vi "picross-complete.vi"() -> ()   [LabVIEW 2020]
panel:
  out "Top":string[](array[string])
  out "Left":string[](array[string])
  out "2D Picture 100":picture
  out "2D Picture 99":picture
  out "2D Picture 98":picture
  out "2D Picture 97":picture
  out "2D Picture 96":picture
  out "2D Picture 95":picture
  out "2D Picture 94":picture
  out "2D Picture 93":picture
  out "2D Picture 92":picture
  out "2D Picture 91":picture
  out "2D Picture 90":picture
  out "2D Picture 89":picture
  out "2D Picture 88":picture
  out "2D Picture 87":picture
  out "2D Picture 86":picture
  out "2D Picture 85":picture
  out "2D Picture 84":picture
  out "2D Picture 83":picture
  out "2D Picture 82":picture
  out "2D Picture 81":picture
  out "2D Picture 80":picture
  out "2D Picture 79":picture
  out "2D Picture 78":picture
  out "2D Picture 77":picture
  out "2D Picture 76":picture
  out "2D Picture 75":picture
  out "2D Picture 74":picture
  out "2D Picture 73":picture
  out "2D Picture 72":picture
  out "2D Picture 71":picture
  out "2D Picture 70":picture
  out "2D Picture 69":picture
  out "2D Picture 68":picture
  out "2D Picture 67":picture
  out "2D Picture 66":picture
  out "2D Picture 65":picture
  out "2D Picture 64":picture
  out "2D Picture 63":picture
  out "2D Picture 62":picture
  out "2D Picture 61":picture
  out "2D Picture 60":picture
  out "2D Picture 59":picture
  out "2D Picture 58":picture
  out "2D Picture 57":picture
  out "2D Picture 56":picture
  out "2D Picture 55":picture
  out "2D Picture 54":picture
  out "2D Picture 53":picture
  out "2D Picture 52":picture
  out "2D Picture 51":picture
  out "2D Picture 50":picture
  out "2D Picture 49":picture
  out "2D Picture 48":picture
  out "2D Picture 47":picture
  out "2D Picture 46":picture
  out "2D Picture 45":picture
  out "2D Picture 44":picture
  out "2D Picture 43":picture
  out "2D Picture 42":picture
  out "2D Picture 41":picture
  out "2D Picture 40":picture
  out "2D Picture 39":picture
  out "2D Picture 38":picture
  out "2D Picture 37":picture
  out "2D Picture 36":picture
  out "2D Picture 35":picture
  out "2D Picture 34":picture
  out "2D Picture 33":picture
  out "2D Picture 32":picture
  out "2D Picture 31":picture
  out "2D Picture 30":picture
  out "2D Picture 29":picture
  out "2D Picture 28":picture
  out "2D Picture 27":picture
  out "2D Picture 26":picture
  out "2D Picture 25":picture
  out "2D Picture 24":picture
  out "2D Picture 23":picture
  out "2D Picture 22":picture
  out "2D Picture 21":picture
  out "2D Picture 20":picture
  out "2D Picture 19":picture
  out "2D Picture 18":picture
  out "2D Picture 17":picture
  out "2D Picture 16":picture
  out "2D Picture 15":picture
  out "2D Picture 14":picture
  out "2D Picture 13":picture
  out "2D Picture 12":picture
  out "2D Picture 11":picture
  out "2D Picture 10":picture
  out "2D Picture 9":picture
  out "2D Picture 8":picture
  out "2D Picture 7":picture
  out "2D Picture 6":picture
  out "2D Picture 5":picture
  out "2D Picture 4":picture
  out "2D Picture 3":picture
  out "2D Picture 2":picture
  out "2D Picture":picture
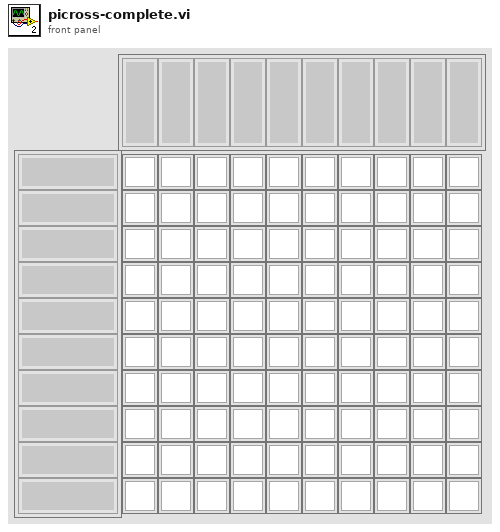
[diagram p1: front panel]
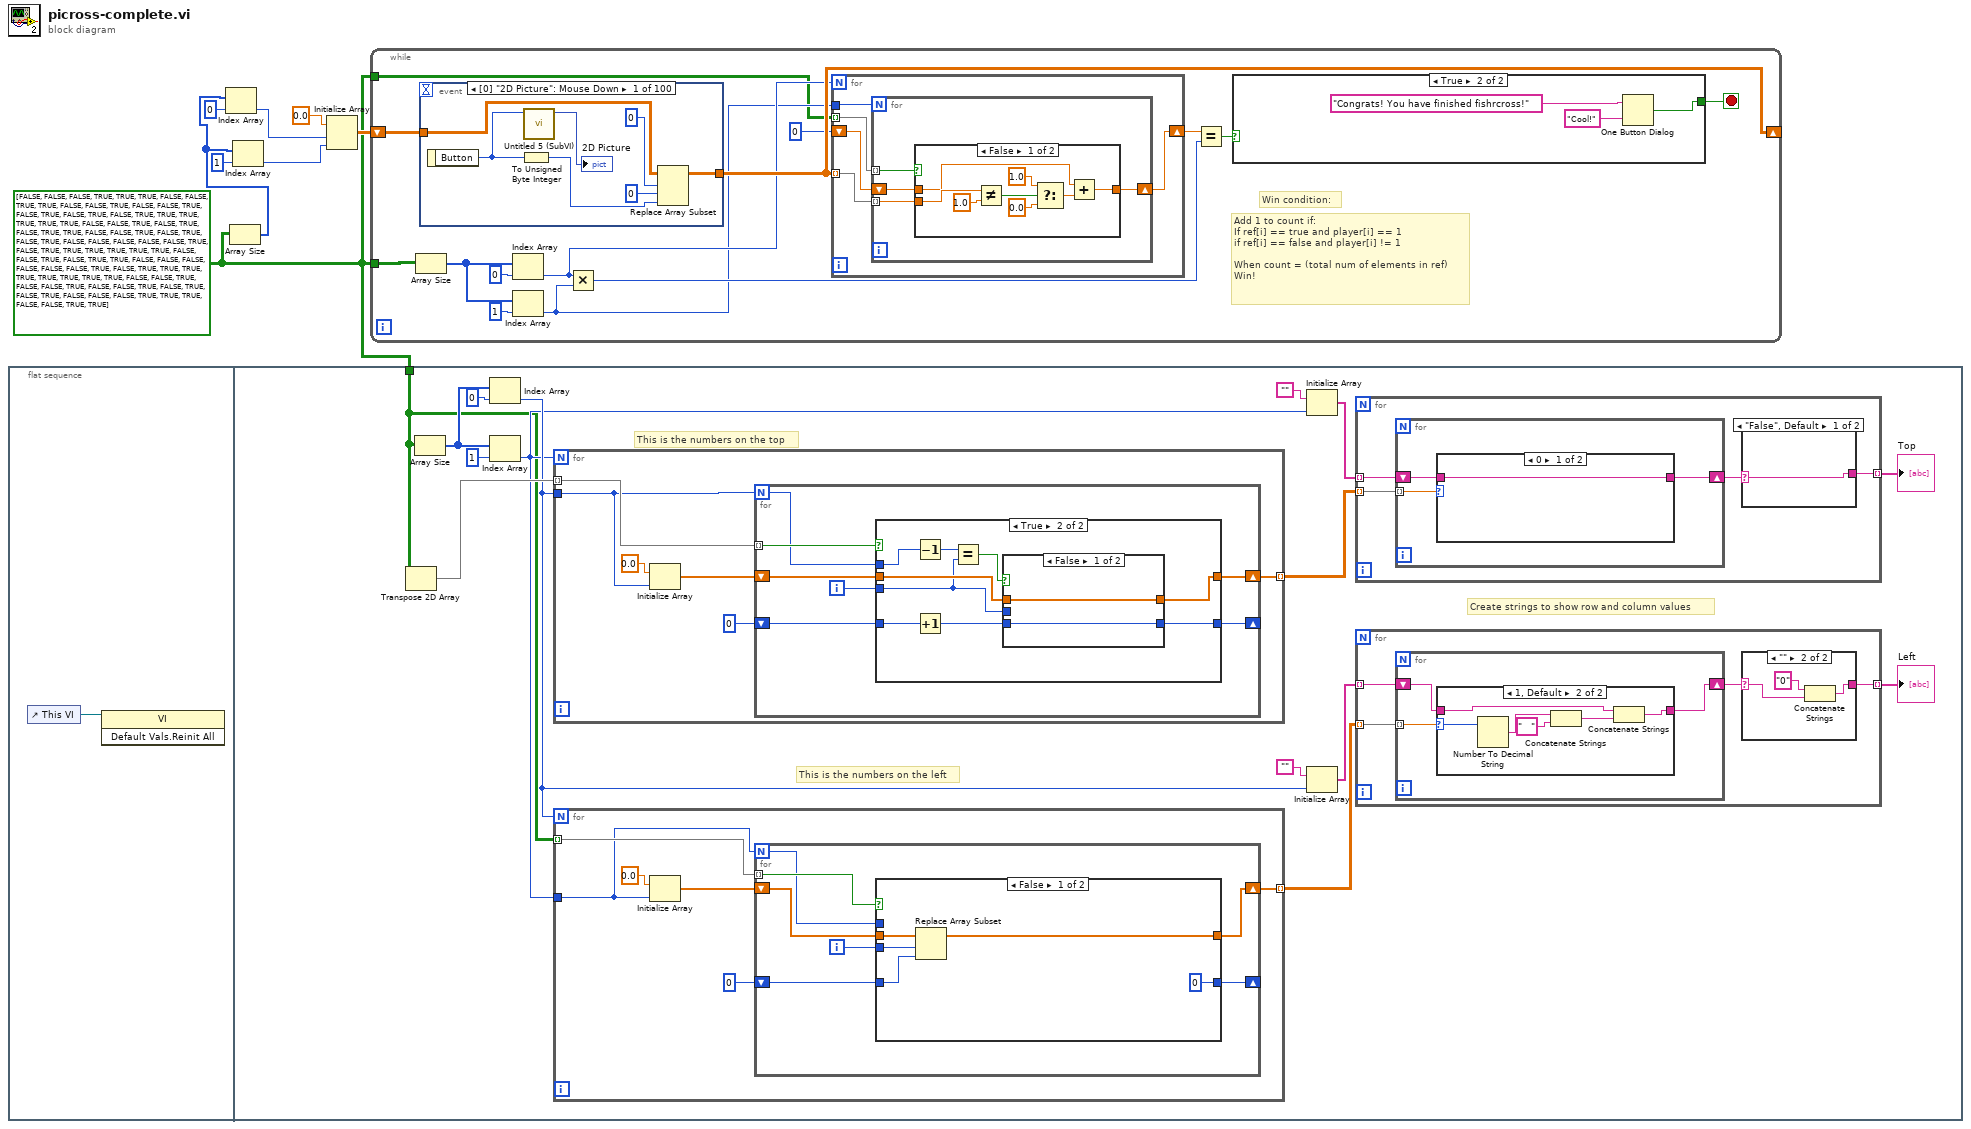
[diagram p0: block diagram]
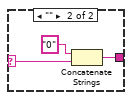
[diagram p2: hidden frame]
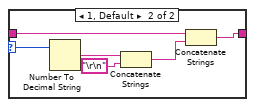
[diagram p3: hidden frame]
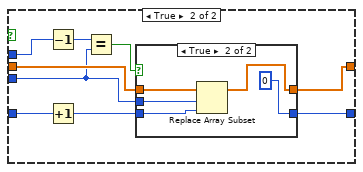
[diagram p6: hidden frame]
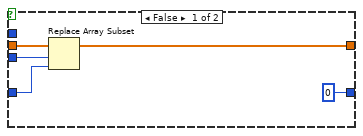
[diagram p8: hidden frame]
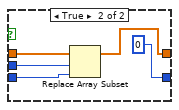
[diagram p9: hidden frame]
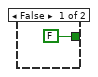
[diagram p10: hidden frame]
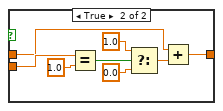
[diagram p11: hidden frame]
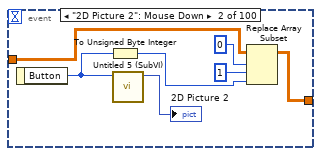
[diagram p12: hidden frame]
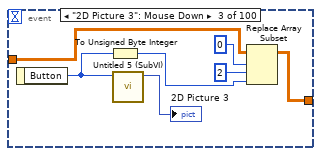
[diagram p13: hidden frame]
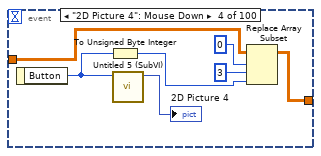
[diagram p14: hidden frame]
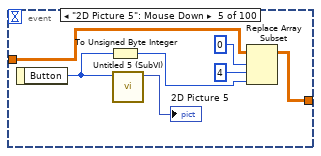
[diagram p15: hidden frame]
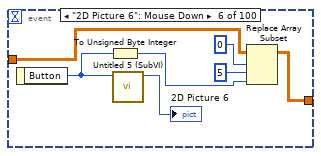
[diagram p16: hidden frame]
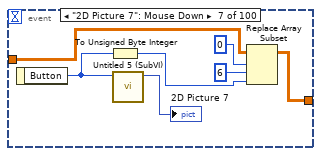
[diagram p17: hidden frame]
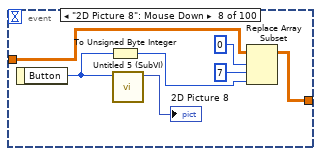
[diagram p18: hidden frame]
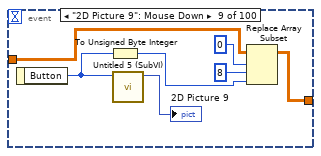
[diagram p19: hidden frame]
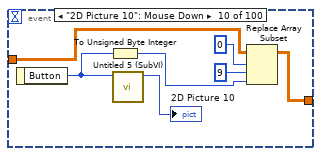
[diagram p20: hidden frame]
diagram:
  w3 = bool[][] [[FALSE, FALSE, FALSE, TRUE, TRUE, TRUE, FALSE, FALSE, TRUE, TRUE], [FALSE, FALSE, TRUE, FALSE, FALSE, TRUE, FALSE, TRUE, FALSE, TRUE], [FALSE, TRUE, TRUE, TRUE, TRUE, TRUE, TRUE, FALSE, FALSE, TRUE], [FALSE, TRUE, FALSE, TRUE, TRUE, FALSE, FALSE, TRUE, FALSE, TRUE], [FALSE, TRUE, FALSE, FALSE, FALSE, FALSE, FALSE, TRUE, FALSE, TRUE], [TRUE, TRUE, TRUE, TRUE, TRUE, FALSE, FALSE, TRUE, FALSE, TRUE], [TRUE, FALSE, FALSE, FALSE, FALSE, FALSE, FALSE, TRUE, FALSE, TRUE], [TRUE, TRUE, TRUE, TRUE, TRUE, TRUE, TRUE, FALSE, FALSE, TRUE], [FALSE, FALSE, TRUE, FALSE, FALSE, TRUE, FALSE, TRUE, FALSE, TRUE], [FALSE, FALSE, FALSE, TRUE, TRUE, TRUE, FALSE, FALSE, TRUE, TRUE]]
  n1 = flat-sequence {
    tunnel: w3 -> [w10]
    frame #0 {
      n2 = control-ref of="This VI"() -> (w9:refnum<vi>)
      n3 = invoke class="VI" method="Default Vals.Reinit All"(reference=w9) -> ()  [unwired: 2 in, 3 out]
    }
    frame #1 {
      # "Create strings to show row and column values"
      # "This is the numbers on the top"
      # "This is the numbers on the left"
      n4 = Transpose 2D Array(2D array=w10) -> (transposed array=w24:bool[][])
      n5 = Array Size(array=w10) -> (size(s)=w23:i32[])
      n6 = Index Array(array=w23, index=0) -> (element=w19:i32)
      n7 = Index Array(array=w23, index=1) -> (element=w14:i32)
      n8 = for {
        N: w14 -> [_]
        tunnel: w19 -> [w95]
        tunnel: w24 -> [w100] mode=indexing
        tunnel: [w96] -> w12 mode=indexing
        n9 = Initialize Array(0.0 ("element"), w95) -> (w97:dbl[])
        n10 = for {
          N: w95 -> [w101]
          tunnel: w100 -> [w107] mode=indexing
          shift-right: [w103] -> w96
          shift-left: w97 -> [w106]
          shift-right: [w104] -> _
          shift-left: 0 -> [w105]
          i -> [w102]
          n11 = case shown="True" w107 {
            tunnel: w106 -> [w111 w114]
            tunnel: w105 -> [w112 w121]
            tunnel: [0 w116] -> w104
            tunnel: [w110 w115] -> w103
            tunnel: w102 -> [w108 w113]
            tunnel: w101 -> [_ w120]
            frame False {
              n12 = Replace Array Subset(array=w111, new element=w112, index=w108) -> (w110:dbl[])
            }
            frame True {
              n13 = Decrement(x=w120) -> (x-1=w119:i32)
              n14 = Increment(x=w121) -> (x+1=w117:i32)
              n15 = Equal?(x=w119, y=w113) -> (x = y?=w118:bool)
              n16 = case shown="False" w118 {
                tunnel: w117 -> [w123 w127]
                tunnel: [w123 0] -> w116
                tunnel: [w122 w126] -> w115
                tunnel: w114 -> [w122 w128]
                tunnel: w113 -> [_ w124]
                frame False {
                }
                frame True {
                  n17 = Replace Array Subset(array=w128, new element=w127, index=w124) -> (w126:dbl[])
                }
              }
            }
          }
        }
      }
      n18 = for {
        N: w19 -> [_]
        tunnel: w14 -> [w61]
        tunnel: w10 -> [w66] mode=indexing
        tunnel: [w62] -> w20 mode=indexing
        n19 = Initialize Array(0.0 ("element"), w61) -> (w63:dbl[])
        n20 = for {
          N: w61 -> [w67]
          tunnel: w66 -> [w73] mode=indexing
          shift-right: [w69] -> w62
          shift-left: w63 -> [w72]
          shift-right: [w70] -> _
          shift-left: 0 -> [w71]
          i -> [w68]
          n21 = case shown="False" w73 {
            tunnel: w72 -> [w77 w80]
            tunnel: w71 -> [w78 w87]
            tunnel: [0 w82] -> w70
            tunnel: [w76 w81] -> w69
            tunnel: w68 -> [w74 w79]
            tunnel: w67 -> [_ w86]
            frame False {
              n22 = Replace Array Subset(array=w77, new element=w78, index=w74) -> (w76:dbl[])
            }
            frame True {
              n23 = Decrement(x=w86) -> (x-1=w85:i32)
              n24 = Increment(x=w87) -> (x+1=w83:i32)
              n25 = Equal?(x=w85, y=w79) -> (x = y?=w84:bool)
              n26 = case shown="True" w84 {
                tunnel: w83 -> [w89 w93]
                tunnel: [w89 0] -> w82
                tunnel: [w88 w92] -> w81
                tunnel: w80 -> [w88 w94]
                tunnel: w79 -> [_ w90]
                frame False {
                }
                frame True {
                  n27 = Replace Array Subset(array=w94, new element=w93, index=w90) -> (w92:dbl[])
                }
              }
            }
          }
        }
      }
      n28 = Initialize Array("", w14) -> (w13:string[])
      n29 = Initialize Array("", w19) -> (w17:string[])
      n30 = for {
        tunnel: w12 -> [w28] mode=indexing
        tunnel: w13 -> [w27] mode=indexing
        tunnel: [w25] -> w11 mode=indexing
        n31 = for {
          tunnel: w28 -> [w35] mode=indexing
          shift-right: [w34] -> w26
          shift-left: w27 -> [w33]
          n32 = case shown="0" w35 {
            selector: w35 -> [_ w42]
            tunnel: [w36 w37] -> w34
            tunnel: w33 -> [w36 w38]
            frame 0 {
            }
            frame 1, Default {
              n33 = Number To Decimal String(number=w42) -> (decimal integer string=w41:string)  [unwired: 1 in]
              n34 = Concatenate Strings(w41, "\r\n") -> (w39:string)
              n35 = Concatenate Strings(w38, w39) -> (w37:string)
            }
          }
        }
        n36 = case shown="\"False\", Default" w26 {
          selector: w26 -> [w29 w31]
          tunnel: [w29 w30] -> w25
          frame "False", Default {
          }
          frame "" {
            n37 = Concatenate Strings("0" ("string"), w31) -> (w30:string)
          }
        }
      }
      "Top" <- w11
      n38 = for {
        tunnel: w20 -> [w46] mode=indexing
        tunnel: w17 -> [w45] mode=indexing
        tunnel: [w43] -> w16 mode=indexing
        n39 = for {
          tunnel: w46 -> [w53] mode=indexing
          shift-right: [w52] -> w44
          shift-left: w45 -> [w51]
          n40 = case shown="1, Default" w53 {
            selector: w53 -> [_ w60]
            tunnel: [w54 w56] -> w52
            tunnel: w51 -> [w54 w57]
            frame 0 {
            }
            frame 1, Default {
              n41 = Number To Decimal String(number=w60) -> (decimal integer string=w59:string)  [unwired: 1 in]
              n42 = Concatenate Strings(w59, "   ") -> (w58:string)
              n43 = Concatenate Strings(w57, w58) -> (w56:string)
            }
          }
        }
        n44 = case shown="\"\"" w44 {
          selector: w44 -> [w47 w49]
          tunnel: [w47 w48] -> w43
          frame "False", Default {
          }
          frame "" {
            n45 = Concatenate Strings("0" ("string"), w49) -> (w48:string)
          }
        }
      }
      "Left" <- w16
    }
  }
  n46 = Array Size(array=w3) -> (size(s)=w2:i32[])
  n47 = Index Array(array=w2, index=0) -> (element=w4:i32)
  n48 = Index Array(array=w2, index=1) -> (element=w1:i32)
  n49 = Initialize Array(0.0 ("element"), w4, w1) -> (w7:dbl[][])
  n50 = while {
    shift-right: [w138] -> _
    shift-left: w7 -> [w142]
    tunnel: w3 -> [w130]
    tunnel: w3 -> [w129]
    stop <- w133 stop-if-true
    # "Add 1 to count if:\nIf ref[i] == true and player[i] == 1\nif ref[i] == false and player[i] != 1\n\nWhen count = (total num of elements in ref)\nWin!"
    # "Win condition:"
    n51 = Array Size(array=w129) -> (size(s)=w141:i32[])
    n52 = event shown="[0] \"2D Picture\": Mouse Down" {
      selector: _ -> [_ _ _ _ _ _ _ _ _ _ _ _ _ _ _ _ _ _ _ _ _ _ _ _ _ _ _ _ _ _ _ _ _ _ _ _ _ _ _ _ _ _ _ _ _ _ _ _ _ _ _ _ _ _ _ _ _ _ _ _ _ _ _ _ _ _ _ _ _ _ _ _ _ _ _ _ _ _ _ _ _ _ _ _ _ _ _ _ _ _ _ _ _ _ _ _ _ _ _ _]
      dyn-events: _ -> [_ _ _ _ _ _ _ _ _ _ _ _ _ _ _ _ _ _ _ _ _ _ _ _ _ _ _ _ _ _ _ _ _ _ _ _ _ _ _ _ _ _ _ _ _ _ _ _ _ _ _ _ _ _ _ _ _ _ _ _ _ _ _ _ _ _ _ _ _ _ _ _ _ _ _ _ _ _ _ _ _ _ _ _ _ _ _ _ _ _ _ _ _ _ _ _ _ _ _ _]
      timeout: _ -> [_ _ _ _ _ _ _ _ _ _ _ _ _ _ _ _ _ _ _ _ _ _ _ _ _ _ _ _ _ _ _ _ _ _ _ _ _ _ _ _ _ _ _ _ _ _ _ _ _ _ _ _ _ _ _ _ _ _ _ _ _ _ _ _ _ _ _ _ _ _ _ _ _ _ _ _ _ _ _ _ _ _ _ _ _ _ _ _ _ _ _ _ _ _ _ _ _ _ _ _]
      tunnel: w142 -> [w176 w183 w190 w197 w204 w211 w218 w225 w232 w239 w246 w253 w260 w267 w274 w281 w288 w295 w302 w309 w316 w323 w330 w337 w344 w351 w358 w365 w372 w379 w386 w393 w400 w407 w414 w421 w428 w435 w442 w449 w456 w463 w470 w477 w484 w491 w498 w505 w512 w519 w526 w533 w540 w547 w554 w561 w568 w575 w582 w589 w596 w603 w610 w617 w624 w631 w638 w645 w652 w659 w666 w673 w680 w687 w694 w701 w708 w715 w722 w729 w736 w743 w750 w757 w764 w771 w778 w785 w792 w799 w806 w813 w820 w827 w834 w841 w848 w855 w862 w869]
      tunnel: [w172 w179 w186 w193 w201 w207 w214 w221 w228 w235 w242 w249 w256 w263 w270 w277 w284 w291 w298 w305 w312 w319 w326 w333 w340 w347 w354 w361 w368 w375 w382 w389 w396 w403 w410 w417 w424 w431 w438 w445 w452 w459 w466 w473 w480 w487 w494 w501 w508 w515 w522 w529 w536 w543 w550 w557 w564 w571 w578 w585 w592 w599 w606 w613 w620 w627 w634 w641 w648 w655 w662 w669 w676 w683 w691 w697 w704 w711 w718 w725 w732 w739 w746 w753 w760 w767 w774 w781 w788 w795 w802 w809 w816 w823 w830 w837 w844 w851 w858 w865] -> w138
      event "2D Picture": Mouse Down {
        n53 = event-data() -> ("Button"=w177:u16)  [unwired: 1 in]
        n54 = To Unsigned Byte Integer(number=w177) -> (unsigned 8bit integer=w173:u8)
        n55 = call "Untitled 5 (SubVI).vi"("Button"=w177) -> ("new picture"=→"2D Picture":picture)  [unwired: 10 in]
        n56 = Replace Array Subset(array=w176, new element=w173, index (row)=0, index (col)=0) -> (w172:dbl[][])
      }
      event "2D Picture 2": Mouse Down {
        n57 = event-data() -> ("Button"=w184:u16)  [unwired: 1 in]
        n58 = To Unsigned Byte Integer(number=w184) -> (unsigned 8bit integer=w180:u8)
        n59 = call "Untitled 5 (SubVI).vi"("Button"=w184) -> ("new picture"=→"2D Picture 2":picture)  [unwired: 10 in]
        n60 = Replace Array Subset(array=w183, new element=w180, index (row)=0, index (col)=1) -> (w179:dbl[][])
      }
      event "2D Picture 3": Mouse Down {
        n61 = event-data() -> ("Button"=w191:u16)  [unwired: 1 in]
        n62 = To Unsigned Byte Integer(number=w191) -> (unsigned 8bit integer=w187:u8)
        n63 = call "Untitled 5 (SubVI).vi"("Button"=w191) -> ("new picture"=→"2D Picture 3":picture)  [unwired: 10 in]
        n64 = Replace Array Subset(array=w190, new element=w187, index (row)=0, index (col)=2) -> (w186:dbl[][])
      }
      event "2D Picture 4": Mouse Down {
        n65 = event-data() -> ("Button"=w198:u16)  [unwired: 1 in]
        n66 = To Unsigned Byte Integer(number=w198) -> (unsigned 8bit integer=w194:u8)
        n67 = call "Untitled 5 (SubVI).vi"("Button"=w198) -> ("new picture"=→"2D Picture 4":picture)  [unwired: 10 in]
        n68 = Replace Array Subset(array=w197, new element=w194, index (row)=0, index (col)=3) -> (w193:dbl[][])
      }
      event "2D Picture 5": Mouse Down {
        n69 = event-data() -> ("Button"=w205:u16)  [unwired: 1 in]
        n70 = To Unsigned Byte Integer(number=w205) -> (unsigned 8bit integer=w202:u8)
        n71 = call "Untitled 5 (SubVI).vi"("Button"=w205) -> ("new picture"=→"2D Picture 5":picture)  [unwired: 10 in]
        n72 = Replace Array Subset(array=w204, new element=w202, index (row)=0, index (col)=4) -> (w201:dbl[][])
      }
      event "2D Picture 6": Mouse Down {
        n73 = event-data() -> ("Button"=w212:u16)  [unwired: 1 in]
        n74 = To Unsigned Byte Integer(number=w212) -> (unsigned 8bit integer=w208:u8)
        n75 = call "Untitled 5 (SubVI).vi"("Button"=w212) -> ("new picture"=→"2D Picture 6":picture)  [unwired: 10 in]
        n76 = Replace Array Subset(array=w211, new element=w208, index (row)=0, index (col)=5) -> (w207:dbl[][])
      }
      event "2D Picture 7": Mouse Down {
        n77 = event-data() -> ("Button"=w219:u16)  [unwired: 1 in]
        n78 = To Unsigned Byte Integer(number=w219) -> (unsigned 8bit integer=w215:u8)
        n79 = call "Untitled 5 (SubVI).vi"("Button"=w219) -> ("new picture"=→"2D Picture 7":picture)  [unwired: 10 in]
        n80 = Replace Array Subset(array=w218, new element=w215, index (row)=0, index (col)=6) -> (w214:dbl[][])
      }
      event "2D Picture 8": Mouse Down {
        n81 = event-data() -> ("Button"=w226:u16)  [unwired: 1 in]
        n82 = To Unsigned Byte Integer(number=w226) -> (unsigned 8bit integer=w222:u8)
        n83 = call "Untitled 5 (SubVI).vi"("Button"=w226) -> ("new picture"=→"2D Picture 8":picture)  [unwired: 10 in]
        n84 = Replace Array Subset(array=w225, new element=w222, index (row)=0, index (col)=7) -> (w221:dbl[][])
      }
      event "2D Picture 9": Mouse Down {
        n85 = event-data() -> ("Button"=w233:u16)  [unwired: 1 in]
        n86 = To Unsigned Byte Integer(number=w233) -> (unsigned 8bit integer=w229:u8)
        n87 = call "Untitled 5 (SubVI).vi"("Button"=w233) -> ("new picture"=→"2D Picture 9":picture)  [unwired: 10 in]
        n88 = Replace Array Subset(array=w232, new element=w229, index (row)=0, index (col)=8) -> (w228:dbl[][])
      }
      event "2D Picture 10": Mouse Down {
        n89 = event-data() -> ("Button"=w240:u16)  [unwired: 1 in]
        n90 = To Unsigned Byte Integer(number=w240) -> (unsigned 8bit integer=w236:u8)
        n91 = call "Untitled 5 (SubVI).vi"("Button"=w240) -> ("new picture"=→"2D Picture 10":picture)  [unwired: 10 in]
        n92 = Replace Array Subset(array=w239, new element=w236, index (row)=0, index (col)=9) -> (w235:dbl[][])
      }
      event "2D Picture 11": Mouse Down {
        n93 = event-data() -> ("Button"=w247:u16)  [unwired: 1 in]
        n94 = To Unsigned Byte Integer(number=w247) -> (unsigned 8bit integer=w243:u8)
        n95 = call "Untitled 5 (SubVI).vi"("Button"=w247) -> ("new picture"=→"2D Picture 11":picture)  [unwired: 10 in]
        n96 = Replace Array Subset(array=w246, new element=w243, index (row)=1, index (col)=0) -> (w242:dbl[][])
      }
      event "2D Picture 12": Mouse Down {
        n97 = event-data() -> ("Button"=w254:u16)  [unwired: 1 in]
        n98 = To Unsigned Byte Integer(number=w254) -> (unsigned 8bit integer=w250:u8)
        n99 = call "Untitled 5 (SubVI).vi"("Button"=w254) -> ("new picture"=→"2D Picture 12":picture)  [unwired: 10 in]
        n100 = Replace Array Subset(array=w253, new element=w250, index (row)=1, index (col)=1) -> (w249:dbl[][])
      }
      event "2D Picture 13": Mouse Down {
        n101 = event-data() -> ("Button"=w261:u16)  [unwired: 1 in]
        n102 = To Unsigned Byte Integer(number=w261) -> (unsigned 8bit integer=w257:u8)
        n103 = call "Untitled 5 (SubVI).vi"("Button"=w261) -> ("new picture"=→"2D Picture 13":picture)  [unwired: 10 in]
        n104 = Replace Array Subset(array=w260, new element=w257, index (row)=1, index (col)=2) -> (w256:dbl[][])
      }
      event "2D Picture 14": Mouse Down {
        n105 = event-data() -> ("Button"=w268:u16)  [unwired: 1 in]
        n106 = To Unsigned Byte Integer(number=w268) -> (unsigned 8bit integer=w264:u8)
        n107 = call "Untitled 5 (SubVI).vi"("Button"=w268) -> ("new picture"=→"2D Picture 14":picture)  [unwired: 10 in]
        n108 = Replace Array Subset(array=w267, new element=w264, index (row)=1, index (col)=3) -> (w263:dbl[][])
      }
      event "2D Picture 15": Mouse Down {
        n109 = event-data() -> ("Button"=w275:u16)  [unwired: 1 in]
        n110 = To Unsigned Byte Integer(number=w275) -> (unsigned 8bit integer=w271:u8)
        n111 = call "Untitled 5 (SubVI).vi"("Button"=w275) -> ("new picture"=→"2D Picture 15":picture)  [unwired: 10 in]
        n112 = Replace Array Subset(array=w274, new element=w271, index (row)=1, index (col)=4) -> (w270:dbl[][])
      }
      event "2D Picture 16": Mouse Down {
        n113 = event-data() -> ("Button"=w282:u16)  [unwired: 1 in]
        n114 = To Unsigned Byte Integer(number=w282) -> (unsigned 8bit integer=w278:u8)
        n115 = call "Untitled 5 (SubVI).vi"("Button"=w282) -> ("new picture"=→"2D Picture 16":picture)  [unwired: 10 in]
        n116 = Replace Array Subset(array=w281, new element=w278, index (row)=1, index (col)=5) -> (w277:dbl[][])
      }
      event "2D Picture 17": Mouse Down {
        n117 = event-data() -> ("Button"=w289:u16)  [unwired: 1 in]
        n118 = To Unsigned Byte Integer(number=w289) -> (unsigned 8bit integer=w285:u8)
        n119 = call "Untitled 5 (SubVI).vi"("Button"=w289) -> ("new picture"=→"2D Picture 17":picture)  [unwired: 10 in]
        n120 = Replace Array Subset(array=w288, new element=w285, index (row)=1, index (col)=6) -> (w284:dbl[][])
      }
      event "2D Picture 18": Mouse Down {
        n121 = event-data() -> ("Button"=w296:u16)  [unwired: 1 in]
        n122 = To Unsigned Byte Integer(number=w296) -> (unsigned 8bit integer=w292:u8)
        n123 = call "Untitled 5 (SubVI).vi"("Button"=w296) -> ("new picture"=→"2D Picture 18":picture)  [unwired: 10 in]
        n124 = Replace Array Subset(array=w295, new element=w292, index (row)=1, index (col)=7) -> (w291:dbl[][])
      }
      event "2D Picture 19": Mouse Down {
        n125 = event-data() -> ("Button"=w303:u16)  [unwired: 1 in]
        n126 = To Unsigned Byte Integer(number=w303) -> (unsigned 8bit integer=w299:u8)
        n127 = call "Untitled 5 (SubVI).vi"("Button"=w303) -> ("new picture"=→"2D Picture 19":picture)  [unwired: 10 in]
        n128 = Replace Array Subset(array=w302, new element=w299, index (row)=1, index (col)=8) -> (w298:dbl[][])
      }
      event "2D Picture 20": Mouse Down {
        n129 = event-data() -> ("Button"=w310:u16)  [unwired: 1 in]
        n130 = To Unsigned Byte Integer(number=w310) -> (unsigned 8bit integer=w306:u8)
        n131 = call "Untitled 5 (SubVI).vi"("Button"=w310) -> ("new picture"=→"2D Picture 20":picture)  [unwired: 10 in]
        n132 = Replace Array Subset(array=w309, new element=w306, index (row)=1, index (col)=9) -> (w305:dbl[][])
      }
      event "2D Picture 21": Mouse Down {
        n133 = event-data() -> ("Button"=w317:u16)  [unwired: 1 in]
        n134 = To Unsigned Byte Integer(number=w317) -> (unsigned 8bit integer=w313:u8)
        n135 = call "Untitled 5 (SubVI).vi"("Button"=w317) -> ("new picture"=→"2D Picture 21":picture)  [unwired: 10 in]
        n136 = Replace Array Subset(array=w316, new element=w313, index (row)=2, index (col)=0) -> (w312:dbl[][])
      }
      event "2D Picture 22": Mouse Down {
        n137 = event-data() -> ("Button"=w324:u16)  [unwired: 1 in]
        n138 = To Unsigned Byte Integer(number=w324) -> (unsigned 8bit integer=w320:u8)
        n139 = call "Untitled 5 (SubVI).vi"("Button"=w324) -> ("new picture"=→"2D Picture 22":picture)  [unwired: 10 in]
        n140 = Replace Array Subset(array=w323, new element=w320, index (row)=2, index (col)=1) -> (w319:dbl[][])
      }
      event "2D Picture 23": Mouse Down {
        n141 = event-data() -> ("Button"=w331:u16)  [unwired: 1 in]
        n142 = To Unsigned Byte Integer(number=w331) -> (unsigned 8bit integer=w327:u8)
        n143 = call "Untitled 5 (SubVI).vi"("Button"=w331) -> ("new picture"=→"2D Picture 23":picture)  [unwired: 10 in]
        n144 = Replace Array Subset(array=w330, new element=w327, index (row)=2, index (col)=2) -> (w326:dbl[][])
      }
      event "2D Picture 24": Mouse Down {
        n145 = event-data() -> ("Button"=w338:u16)  [unwired: 1 in]
        n146 = To Unsigned Byte Integer(number=w338) -> (unsigned 8bit integer=w334:u8)
        n147 = call "Untitled 5 (SubVI).vi"("Button"=w338) -> ("new picture"=→"2D Picture 24":picture)  [unwired: 10 in]
        n148 = Replace Array Subset(array=w337, new element=w334, index (row)=2, index (col)=3) -> (w333:dbl[][])
      }
      event "2D Picture 25": Mouse Down {
        n149 = event-data() -> ("Button"=w345:u16)  [unwired: 1 in]
        n150 = To Unsigned Byte Integer(number=w345) -> (unsigned 8bit integer=w341:u8)
        n151 = call "Untitled 5 (SubVI).vi"("Button"=w345) -> ("new picture"=→"2D Picture 25":picture)  [unwired: 10 in]
        n152 = Replace Array Subset(array=w344, new element=w341, index (row)=2, index (col)=4) -> (w340:dbl[][])
      }
      event "2D Picture 26": Mouse Down {
        n153 = event-data() -> ("Button"=w352:u16)  [unwired: 1 in]
        n154 = To Unsigned Byte Integer(number=w352) -> (unsigned 8bit integer=w348:u8)
        n155 = call "Untitled 5 (SubVI).vi"("Button"=w352) -> ("new picture"=→"2D Picture 26":picture)  [unwired: 10 in]
        n156 = Replace Array Subset(array=w351, new element=w348, index (row)=2, index (col)=5) -> (w347:dbl[][])
      }
      event "2D Picture 27": Mouse Down {
        n157 = event-data() -> ("Button"=w359:u16)  [unwired: 1 in]
        n158 = To Unsigned Byte Integer(number=w359) -> (unsigned 8bit integer=w355:u8)
        n159 = call "Untitled 5 (SubVI).vi"("Button"=w359) -> ("new picture"=→"2D Picture 27":picture)  [unwired: 10 in]
        n160 = Replace Array Subset(array=w358, new element=w355, index (row)=2, index (col)=6) -> (w354:dbl[][])
      }
      event "2D Picture 28": Mouse Down {
        n161 = event-data() -> ("Button"=w366:u16)  [unwired: 1 in]
        n162 = To Unsigned Byte Integer(number=w366) -> (unsigned 8bit integer=w362:u8)
        n163 = call "Untitled 5 (SubVI).vi"("Button"=w366) -> ("new picture"=→"2D Picture 28":picture)  [unwired: 10 in]
        n164 = Replace Array Subset(array=w365, new element=w362, index (row)=2, index (col)=7) -> (w361:dbl[][])
      }
      event "2D Picture 29": Mouse Down {
        n165 = event-data() -> ("Button"=w373:u16)  [unwired: 1 in]
        n166 = To Unsigned Byte Integer(number=w373) -> (unsigned 8bit integer=w369:u8)
        n167 = call "Untitled 5 (SubVI).vi"("Button"=w373) -> ("new picture"=→"2D Picture 29":picture)  [unwired: 10 in]
        n168 = Replace Array Subset(array=w372, new element=w369, index (row)=2, index (col)=8) -> (w368:dbl[][])
      }
      event "2D Picture 30": Mouse Down {
        n169 = event-data() -> ("Button"=w380:u16)  [unwired: 1 in]
        n170 = To Unsigned Byte Integer(number=w380) -> (unsigned 8bit integer=w376:u8)
        n171 = call "Untitled 5 (SubVI).vi"("Button"=w380) -> ("new picture"=→"2D Picture 30":picture)  [unwired: 10 in]
        n172 = Replace Array Subset(array=w379, new element=w376, index (row)=2, index (col)=9) -> (w375:dbl[][])
      }
      event "2D Picture 31": Mouse Down {
        n173 = event-data() -> ("Button"=w387:u16)  [unwired: 1 in]
        n174 = To Unsigned Byte Integer(number=w387) -> (unsigned 8bit integer=w383:u8)
        n175 = call "Untitled 5 (SubVI).vi"("Button"=w387) -> ("new picture"=→"2D Picture 31":picture)  [unwired: 10 in]
        n176 = Replace Array Subset(array=w386, new element=w383, index (row)=3, index (col)=0) -> (w382:dbl[][])
      }
      event "2D Picture 32": Mouse Down {
        n177 = event-data() -> ("Button"=w394:u16)  [unwired: 1 in]
        n178 = To Unsigned Byte Integer(number=w394) -> (unsigned 8bit integer=w390:u8)
        n179 = call "Untitled 5 (SubVI).vi"("Button"=w394) -> ("new picture"=→"2D Picture 32":picture)  [unwired: 10 in]
        n180 = Replace Array Subset(array=w393, new element=w390, index (row)=3, index (col)=1) -> (w389:dbl[][])
      }
      event "2D Picture 33": Mouse Down {
        n181 = event-data() -> ("Button"=w401:u16)  [unwired: 1 in]
        n182 = To Unsigned Byte Integer(number=w401) -> (unsigned 8bit integer=w397:u8)
        n183 = call "Untitled 5 (SubVI).vi"("Button"=w401) -> ("new picture"=→"2D Picture 33":picture)  [unwired: 10 in]
        n184 = Replace Array Subset(array=w400, new element=w397, index (row)=3, index (col)=2) -> (w396:dbl[][])
      }
      event "2D Picture 34": Mouse Down {
        n185 = event-data() -> ("Button"=w408:u16)  [unwired: 1 in]
        n186 = To Unsigned Byte Integer(number=w408) -> (unsigned 8bit integer=w404:u8)
        n187 = call "Untitled 5 (SubVI).vi"("Button"=w408) -> ("new picture"=→"2D Picture 34":picture)  [unwired: 10 in]
        n188 = Replace Array Subset(array=w407, new element=w404, index (row)=3, index (col)=3) -> (w403:dbl[][])
      }
      event "2D Picture 35": Mouse Down {
        n189 = event-data() -> ("Button"=w415:u16)  [unwired: 1 in]
        n190 = To Unsigned Byte Integer(number=w415) -> (unsigned 8bit integer=w411:u8)
        n191 = call "Untitled 5 (SubVI).vi"("Button"=w415) -> ("new picture"=→"2D Picture 35":picture)  [unwired: 10 in]
        n192 = Replace Array Subset(array=w414, new element=w411, index (row)=3, index (col)=4) -> (w410:dbl[][])
      }
      event "2D Picture 36": Mouse Down {
        n193 = event-data() -> ("Button"=w422:u16)  [unwired: 1 in]
        n194 = To Unsigned Byte Integer(number=w422) -> (unsigned 8bit integer=w418:u8)
        n195 = call "Untitled 5 (SubVI).vi"("Button"=w422) -> ("new picture"=→"2D Picture 36":picture)  [unwired: 10 in]
        n196 = Replace Array Subset(array=w421, new element=w418, index (row)=3, index (col)=5) -> (w417:dbl[][])
      }
      event "2D Picture 37": Mouse Down {
        n197 = event-data() -> ("Button"=w429:u16)  [unwired: 1 in]
        n198 = To Unsigned Byte Integer(number=w429) -> (unsigned 8bit integer=w425:u8)
        n199 = call "Untitled 5 (SubVI).vi"("Button"=w429) -> ("new picture"=→"2D Picture 37":picture)  [unwired: 10 in]
        n200 = Replace Array Subset(array=w428, new element=w425, index (row)=3, index (col)=6) -> (w424:dbl[][])
      }
      event "2D Picture 38": Mouse Down {
        n201 = event-data() -> ("Button"=w436:u16)  [unwired: 1 in]
        n202 = To Unsigned Byte Integer(number=w436) -> (unsigned 8bit integer=w432:u8)
        n203 = call "Untitled 5 (SubVI).vi"("Button"=w436) -> ("new picture"=→"2D Picture 38":picture)  [unwired: 10 in]
        n204 = Replace Array Subset(array=w435, new element=w432, index (row)=3, index (col)=7) -> (w431:dbl[][])
      }
      event "2D Picture 39": Mouse Down {
        n205 = event-data() -> ("Button"=w443:u16)  [unwired: 1 in]
        n206 = To Unsigned Byte Integer(number=w443) -> (unsigned 8bit integer=w439:u8)
        n207 = call "Untitled 5 (SubVI).vi"("Button"=w443) -> ("new picture"=→"2D Picture 39":picture)  [unwired: 10 in]
        n208 = Replace Array Subset(array=w442, new element=w439, index (row)=3, index (col)=8) -> (w438:dbl[][])
      }
      event "2D Picture 40": Mouse Down {
        n209 = event-data() -> ("Button"=w450:u16)  [unwired: 1 in]
        n210 = To Unsigned Byte Integer(number=w450) -> (unsigned 8bit integer=w446:u8)
        n211 = call "Untitled 5 (SubVI).vi"("Button"=w450) -> ("new picture"=→"2D Picture 40":picture)  [unwired: 10 in]
        n212 = Replace Array Subset(array=w449, new element=w446, index (row)=3, index (col)=9) -> (w445:dbl[][])
      }
      event "2D Picture 41": Mouse Down {
        n213 = event-data() -> ("Button"=w457:u16)  [unwired: 1 in]
        n214 = To Unsigned Byte Integer(number=w457) -> (unsigned 8bit integer=w453:u8)
        n215 = call "Untitled 5 (SubVI).vi"("Button"=w457) -> ("new picture"=→"2D Picture 41":picture)  [unwired: 10 in]
        n216 = Replace Array Subset(array=w456, new element=w453, index (row)=4, index (col)=0) -> (w452:dbl[][])
      }
      event "2D Picture 42": Mouse Down {
        n217 = event-data() -> ("Button"=w464:u16)  [unwired: 1 in]
        n218 = To Unsigned Byte Integer(number=w464) -> (unsigned 8bit integer=w460:u8)
        n219 = call "Untitled 5 (SubVI).vi"("Button"=w464) -> ("new picture"=→"2D Picture 42":picture)  [unwired: 10 in]
        n220 = Replace Array Subset(array=w463, new element=w460, index (row)=4, index (col)=1) -> (w459:dbl[][])
      }
      event "2D Picture 43": Mouse Down {
        n221 = event-data() -> ("Button"=w471:u16)  [unwired: 1 in]
        n222 = To Unsigned Byte Integer(number=w471) -> (unsigned 8bit integer=w467:u8)
        n223 = call "Untitled 5 (SubVI).vi"("Button"=w471) -> ("new picture"=→"2D Picture 43":picture)  [unwired: 10 in]
        n224 = Replace Array Subset(array=w470, new element=w467, index (row)=4, index (col)=2) -> (w466:dbl[][])
      }
      event "2D Picture 44": Mouse Down {
        n225 = event-data() -> ("Button"=w478:u16)  [unwired: 1 in]
        n226 = To Unsigned Byte Integer(number=w478) -> (unsigned 8bit integer=w474:u8)
        n227 = call "Untitled 5 (SubVI).vi"("Button"=w478) -> ("new picture"=→"2D Picture 44":picture)  [unwired: 10 in]
        n228 = Replace Array Subset(array=w477, new element=w474, index (row)=4, index (col)=3) -> (w473:dbl[][])
      }
      event "2D Picture 45": Mouse Down {
        n229 = event-data() -> ("Button"=w485:u16)  [unwired: 1 in]
        n230 = To Unsigned Byte Integer(number=w485) -> (unsigned 8bit integer=w481:u8)
        n231 = call "Untitled 5 (SubVI).vi"("Button"=w485) -> ("new picture"=→"2D Picture 45":picture)  [unwired: 10 in]
        n232 = Replace Array Subset(array=w484, new element=w481, index (row)=4, index (col)=4) -> (w480:dbl[][])
      }
      event "2D Picture 46": Mouse Down {
        n233 = event-data() -> ("Button"=w492:u16)  [unwired: 1 in]
        n234 = To Unsigned Byte Integer(number=w492) -> (unsigned 8bit integer=w488:u8)
        n235 = call "Untitled 5 (SubVI).vi"("Button"=w492) -> ("new picture"=→"2D Picture 46":picture)  [unwired: 10 in]
        n236 = Replace Array Subset(array=w491, new element=w488, index (row)=4, index (col)=5) -> (w487:dbl[][])
      }
      event "2D Picture 47": Mouse Down {
        n237 = event-data() -> ("Button"=w499:u16)  [unwired: 1 in]
        n238 = To Unsigned Byte Integer(number=w499) -> (unsigned 8bit integer=w495:u8)
        n239 = call "Untitled 5 (SubVI).vi"("Button"=w499) -> ("new picture"=→"2D Picture 47":picture)  [unwired: 10 in]
        n240 = Replace Array Subset(array=w498, new element=w495, index (row)=4, index (col)=6) -> (w494:dbl[][])
      }
      event "2D Picture 48": Mouse Down {
        n241 = event-data() -> ("Button"=w506:u16)  [unwired: 1 in]
        n242 = To Unsigned Byte Integer(number=w506) -> (unsigned 8bit integer=w502:u8)
        n243 = call "Untitled 5 (SubVI).vi"("Button"=w506) -> ("new picture"=→"2D Picture 48":picture)  [unwired: 10 in]
        n244 = Replace Array Subset(array=w505, new element=w502, index (row)=4, index (col)=7) -> (w501:dbl[][])
      }
      event "2D Picture 49": Mouse Down {
        n245 = event-data() -> ("Button"=w513:u16)  [unwired: 1 in]
        n246 = To Unsigned Byte Integer(number=w513) -> (unsigned 8bit integer=w509:u8)
        n247 = call "Untitled 5 (SubVI).vi"("Button"=w513) -> ("new picture"=→"2D Picture 49":picture)  [unwired: 10 in]
        n248 = Replace Array Subset(array=w512, new element=w509, index (row)=4, index (col)=8) -> (w508:dbl[][])
      }
      event "2D Picture 50": Mouse Down {
        n249 = event-data() -> ("Button"=w520:u16)  [unwired: 1 in]
        n250 = To Unsigned Byte Integer(number=w520) -> (unsigned 8bit integer=w516:u8)
        n251 = call "Untitled 5 (SubVI).vi"("Button"=w520) -> ("new picture"=→"2D Picture 50":picture)  [unwired: 10 in]
        n252 = Replace Array Subset(array=w519, new element=w516, index (row)=4, index (col)=9) -> (w515:dbl[][])
      }
      event "2D Picture 51": Mouse Down {
        n253 = event-data() -> ("Button"=w527:u16)  [unwired: 1 in]
        n254 = To Unsigned Byte Integer(number=w527) -> (unsigned 8bit integer=w523:u8)
        n255 = call "Untitled 5 (SubVI).vi"("Button"=w527) -> ("new picture"=→"2D Picture 51":picture)  [unwired: 10 in]
        n256 = Replace Array Subset(array=w526, new element=w523, index (row)=5, index (col)=0) -> (w522:dbl[][])
      }
      event "2D Picture 52": Mouse Down {
        n257 = event-data() -> ("Button"=w534:u16)  [unwired: 1 in]
        n258 = To Unsigned Byte Integer(number=w534) -> (unsigned 8bit integer=w530:u8)
        n259 = call "Untitled 5 (SubVI).vi"("Button"=w534) -> ("new picture"=→"2D Picture 52":picture)  [unwired: 10 in]
        n260 = Replace Array Subset(array=w533, new element=w530, index (row)=5, index (col)=1) -> (w529:dbl[][])
      }
      event "2D Picture 53": Mouse Down {
        n261 = event-data() -> ("Button"=w541:u16)  [unwired: 1 in]
        n262 = To Unsigned Byte Integer(number=w541) -> (unsigned 8bit integer=w537:u8)
        n263 = call "Untitled 5 (SubVI).vi"("Button"=w541) -> ("new picture"=→"2D Picture 53":picture)  [unwired: 10 in]
        n264 = Replace Array Subset(array=w540, new element=w537, index (row)=5, index (col)=2) -> (w536:dbl[][])
      }
      event "2D Picture 54": Mouse Down {
        n265 = event-data() -> ("Button"=w548:u16)  [unwired: 1 in]
        n266 = To Unsigned Byte Integer(number=w548) -> (unsigned 8bit integer=w544:u8)
        n267 = call "Untitled 5 (SubVI).vi"("Button"=w548) -> ("new picture"=→"2D Picture 54":picture)  [unwired: 10 in]
        n268 = Replace Array Subset(array=w547, new element=w544, index (row)=5, index (col)=3) -> (w543:dbl[][])
      }
      event "2D Picture 55": Mouse Down {
        n269 = event-data() -> ("Button"=w555:u16)  [unwired: 1 in]
        n270 = To Unsigned Byte Integer(number=w555) -> (unsigned 8bit integer=w551:u8)
        n271 = call "Untitled 5 (SubVI).vi"("Button"=w555) -> ("new picture"=→"2D Picture 55":picture)  [unwired: 10 in]
        n272 = Replace Array Subset(array=w554, new element=w551, index (row)=5, index (col)=4) -> (w550:dbl[][])
      }
      event "2D Picture 56": Mouse Down {
        n273 = event-data() -> ("Button"=w562:u16)  [unwired: 1 in]
        n274 = To Unsigned Byte Integer(number=w562) -> (unsigned 8bit integer=w558:u8)
        n275 = call "Untitled 5 (SubVI).vi"("Button"=w562) -> ("new picture"=→"2D Picture 56":picture)  [unwired: 10 in]
        n276 = Replace Array Subset(array=w561, new element=w558, index (row)=5, index (col)=5) -> (w557:dbl[][])
      }
      event "2D Picture 57": Mouse Down {
        n277 = event-data() -> ("Button"=w569:u16)  [unwired: 1 in]
        n278 = To Unsigned Byte Integer(number=w569) -> (unsigned 8bit integer=w565:u8)
        n279 = call "Untitled 5 (SubVI).vi"("Button"=w569) -> ("new picture"=→"2D Picture 57":picture)  [unwired: 10 in]
        n280 = Replace Array Subset(array=w568, new element=w565, index (row)=5, index (col)=6) -> (w564:dbl[][])
      }
      event "2D Picture 58": Mouse Down {
        n281 = event-data() -> ("Button"=w576:u16)  [unwired: 1 in]
        n282 = To Unsigned Byte Integer(number=w576) -> (unsigned 8bit integer=w572:u8)
        n283 = call "Untitled 5 (SubVI).vi"("Button"=w576) -> ("new picture"=→"2D Picture 58":picture)  [unwired: 10 in]
        n284 = Replace Array Subset(array=w575, new element=w572, index (row)=5, index (col)=7) -> (w571:dbl[][])
      }
      event "2D Picture 59": Mouse Down {
        n285 = event-data() -> ("Button"=w583:u16)  [unwired: 1 in]
        n286 = To Unsigned Byte Integer(number=w583) -> (unsigned 8bit integer=w579:u8)
        n287 = call "Untitled 5 (SubVI).vi"("Button"=w583) -> ("new picture"=→"2D Picture 59":picture)  [unwired: 10 in]
        n288 = Replace Array Subset(array=w582, new element=w579, index (row)=5, index (col)=8) -> (w578:dbl[][])
      }
      event "2D Picture 60": Mouse Down {
        n289 = event-data() -> ("Button"=w590:u16)  [unwired: 1 in]
        n290 = To Unsigned Byte Integer(number=w590) -> (unsigned 8bit integer=w586:u8)
        n291 = call "Untitled 5 (SubVI).vi"("Button"=w590) -> ("new picture"=→"2D Picture 60":picture)  [unwired: 10 in]
        n292 = Replace Array Subset(array=w589, new element=w586, index (row)=5, index (col)=9) -> (w585:dbl[][])
      }
      event "2D Picture 61": Mouse Down {
        n293 = event-data() -> ("Button"=w597:u16)  [unwired: 1 in]
        n294 = To Unsigned Byte Integer(number=w597) -> (unsigned 8bit integer=w593:u8)
        n295 = call "Untitled 5 (SubVI).vi"("Button"=w597) -> ("new picture"=→"2D Picture 61":picture)  [unwired: 10 in]
        n296 = Replace Array Subset(array=w596, new element=w593, index (row)=6, index (col)=0) -> (w592:dbl[][])
      }
      event "2D Picture 62": Mouse Down {
        n297 = event-data() -> ("Button"=w604:u16)  [unwired: 1 in]
        n298 = To Unsigned Byte Integer(number=w604) -> (unsigned 8bit integer=w600:u8)
        n299 = call "Untitled 5 (SubVI).vi"("Button"=w604) -> ("new picture"=→"2D Picture 62":picture)  [unwired: 10 in]
        n300 = Replace Array Subset(array=w603, new element=w600, index (row)=6, index (col)=1) -> (w599:dbl[][])
      }
      event "2D Picture 63": Mouse Down {
        n301 = event-data() -> ("Button"=w611:u16)  [unwired: 1 in]
        n302 = To Unsigned Byte Integer(number=w611) -> (unsigned 8bit integer=w607:u8)
        n303 = call "Untitled 5 (SubVI).vi"("Button"=w611) -> ("new picture"=→"2D Picture 63":picture)  [unwired: 10 in]
        n304 = Replace Array Subset(array=w610, new element=w607, index (row)=6, index (col)=2) -> (w606:dbl[][])
      }
      event "2D Picture 64": Mouse Down {
        n305 = event-data() -> ("Button"=w618:u16)  [unwired: 1 in]
        n306 = To Unsigned Byte Integer(number=w618) -> (unsigned 8bit integer=w614:u8)
        n307 = call "Untitled 5 (SubVI).vi"("Button"=w618) -> ("new picture"=→"2D Picture 64":picture)  [unwired: 10 in]
        n308 = Replace Array Subset(array=w617, new element=w614, index (row)=6, index (col)=3) -> (w613:dbl[][])
      }
      event "2D Picture 65": Mouse Down {
        n309 = event-data() -> ("Button"=w625:u16)  [unwired: 1 in]
        n310 = To Unsigned Byte Integer(number=w625) -> (unsigned 8bit integer=w621:u8)
        n311 = call "Untitled 5 (SubVI).vi"("Button"=w625) -> ("new picture"=→"2D Picture 65":picture)  [unwired: 10 in]
        n312 = Replace Array Subset(array=w624, new element=w621, index (row)=6, index (col)=4) -> (w620:dbl[][])
      }
      event "2D Picture 66": Mouse Down {
        n313 = event-data() -> ("Button"=w632:u16)  [unwired: 1 in]
        n314 = To Unsigned Byte Integer(number=w632) -> (unsigned 8bit integer=w628:u8)
        n315 = call "Untitled 5 (SubVI).vi"("Button"=w632) -> ("new picture"=→"2D Picture 66":picture)  [unwired: 10 in]
        n316 = Replace Array Subset(array=w631, new element=w628, index (row)=6, index (col)=5) -> (w627:dbl[][])
      }
      event "2D Picture 67": Mouse Down {
        n317 = event-data() -> ("Button"=w639:u16)  [unwired: 1 in]
        n318 = To Unsigned Byte Integer(number=w639) -> (unsigned 8bit integer=w635:u8)
        n319 = call "Untitled 5 (SubVI).vi"("Button"=w639) -> ("new picture"=→"2D Picture 67":picture)  [unwired: 10 in]
        n320 = Replace Array Subset(array=w638, new element=w635, index (row)=6, index (col)=6) -> (w634:dbl[][])
      }
      event "2D Picture 68": Mouse Down {
        n321 = event-data() -> ("Button"=w646:u16)  [unwired: 1 in]
        n322 = To Unsigned Byte Integer(number=w646) -> (unsigned 8bit integer=w642:u8)
        n323 = call "Untitled 5 (SubVI).vi"("Button"=w646) -> ("new picture"=→"2D Picture 68":picture)  [unwired: 10 in]
        n324 = Replace Array Subset(array=w645, new element=w642, index (row)=6, index (col)=7) -> (w641:dbl[][])
      }
      event "2D Picture 69": Mouse Down {
        n325 = event-data() -> ("Button"=w653:u16)  [unwired: 1 in]
        n326 = To Unsigned Byte Integer(number=w653) -> (unsigned 8bit integer=w649:u8)
        n327 = call "Untitled 5 (SubVI).vi"("Button"=w653) -> ("new picture"=→"2D Picture 69":picture)  [unwired: 10 in]
        n328 = Replace Array Subset(array=w652, new element=w649, index (row)=6, index (col)=8) -> (w648:dbl[][])
      }
      event "2D Picture 70": Mouse Down {
        n329 = event-data() -> ("Button"=w660:u16)  [unwired: 1 in]
        n330 = To Unsigned Byte Integer(number=w660) -> (unsigned 8bit integer=w656:u8)
        n331 = call "Untitled 5 (SubVI).vi"("Button"=w660) -> ("new picture"=→"2D Picture 70":picture)  [unwired: 10 in]
        n332 = Replace Array Subset(array=w659, new element=w656, index (row)=6, index (col)=9) -> (w655:dbl[][])
      }
      event "2D Picture 71": Mouse Down {
        n333 = event-data() -> ("Button"=w667:u16)  [unwired: 1 in]
        n334 = To Unsigned Byte Integer(number=w667) -> (unsigned 8bit integer=w663:u8)
        n335 = call "Untitled 5 (SubVI).vi"("Button"=w667) -> ("new picture"=→"2D Picture 71":picture)  [unwired: 10 in]
        n336 = Replace Array Subset(array=w666, new element=w663, index (row)=7, index (col)=0) -> (w662:dbl[][])
      }
      event "2D Picture 72": Mouse Down {
        n337 = event-data() -> ("Button"=w674:u16)  [unwired: 1 in]
        n338 = To Unsigned Byte Integer(number=w674) -> (unsigned 8bit integer=w670:u8)
        n339 = call "Untitled 5 (SubVI).vi"("Button"=w674) -> ("new picture"=→"2D Picture 72":picture)  [unwired: 10 in]
        n340 = Replace Array Subset(array=w673, new element=w670, index (row)=7, index (col)=1) -> (w669:dbl[][])
      }
      event "2D Picture 73": Mouse Down {
        n341 = event-data() -> ("Button"=w681:u16)  [unwired: 1 in]
        n342 = To Unsigned Byte Integer(number=w681) -> (unsigned 8bit integer=w677:u8)
        n343 = call "Untitled 5 (SubVI).vi"("Button"=w681) -> ("new picture"=→"2D Picture 73":picture)  [unwired: 10 in]
        n344 = Replace Array Subset(array=w680, new element=w677, index (row)=7, index (col)=2) -> (w676:dbl[][])
      }
      event "2D Picture 74": Mouse Down {
        n345 = event-data() -> ("Button"=w688:u16)  [unwired: 1 in]
        n346 = To Unsigned Byte Integer(number=w688) -> (unsigned 8bit integer=w684:u8)
        n347 = call "Untitled 5 (SubVI).vi"("Button"=w688) -> ("new picture"=→"2D Picture 74":picture)  [unwired: 10 in]
        n348 = Replace Array Subset(array=w687, new element=w684, index (row)=7, index (col)=3) -> (w683:dbl[][])
      }
      event "2D Picture 75": Mouse Down {
        n349 = event-data() -> ("Button"=w695:u16)  [unwired: 1 in]
        n350 = To Unsigned Byte Integer(number=w695) -> (unsigned 8bit integer=w692:u8)
        n351 = call "Untitled 5 (SubVI).vi"("Button"=w695) -> ("new picture"=→"2D Picture 75":picture)  [unwired: 10 in]
        n352 = Replace Array Subset(array=w694, new element=w692, index (row)=7, index (col)=4) -> (w691:dbl[][])
      }
      event "2D Picture 76": Mouse Down {
        n353 = event-data() -> ("Button"=w702:u16)  [unwired: 1 in]
        n354 = To Unsigned Byte Integer(number=w702) -> (unsigned 8bit integer=w698:u8)
        n355 = call "Untitled 5 (SubVI).vi"("Button"=w702) -> ("new picture"=→"2D Picture 76":picture)  [unwired: 10 in]
        n356 = Replace Array Subset(array=w701, new element=w698, index (row)=7, index (col)=5) -> (w697:dbl[][])
      }
      event "2D Picture 77": Mouse Down {
        n357 = event-data() -> ("Button"=w709:u16)  [unwired: 1 in]
        n358 = To Unsigned Byte Integer(number=w709) -> (unsigned 8bit integer=w705:u8)
        n359 = call "Untitled 5 (SubVI).vi"("Button"=w709) -> ("new picture"=→"2D Picture 77":picture)  [unwired: 10 in]
        n360 = Replace Array Subset(array=w708, new element=w705, index (row)=7, index (col)=6) -> (w704:dbl[][])
      }
      event "2D Picture 78": Mouse Down {
        n361 = event-data() -> ("Button"=w716:u16)  [unwired: 1 in]
        n362 = To Unsigned Byte Integer(number=w716) -> (unsigned 8bit integer=w712:u8)
        n363 = call "Untitled 5 (SubVI).vi"("Button"=w716) -> ("new picture"=→"2D Picture 78":picture)  [unwired: 10 in]
        n364 = Replace Array Subset(array=w715, new element=w712, index (row)=7, index (col)=7) -> (w711:dbl[][])
      }
      event "2D Picture 79": Mouse Down {
        n365 = event-data() -> ("Button"=w723:u16)  [unwired: 1 in]
        n366 = To Unsigned Byte Integer(number=w723) -> (unsigned 8bit integer=w719:u8)
        n367 = call "Untitled 5 (SubVI).vi"("Button"=w723) -> ("new picture"=→"2D Picture 79":picture)  [unwired: 10 in]
        n368 = Replace Array Subset(array=w722, new element=w719, index (row)=7, index (col)=8) -> (w718:dbl[][])
      }
      event "2D Picture 80": Mouse Down {
        n369 = event-data() -> ("Button"=w730:u16)  [unwired: 1 in]
        n370 = To Unsigned Byte Integer(number=w730) -> (unsigned 8bit integer=w726:u8)
        n371 = call "Untitled 5 (SubVI).vi"("Button"=w730) -> ("new picture"=→"2D Picture 80":picture)  [unwired: 10 in]
        n372 = Replace Array Subset(array=w729, new element=w726, index (row)=7, index (col)=9) -> (w725:dbl[][])
      }
      event "2D Picture 81": Mouse Down {
        n373 = event-data() -> ("Button"=w737:u16)  [unwired: 1 in]
        n374 = To Unsigned Byte Integer(number=w737) -> (unsigned 8bit integer=w733:u8)
        n375 = call "Untitled 5 (SubVI).vi"("Button"=w737) -> ("new picture"=→"2D Picture 81":picture)  [unwired: 10 in]
        n376 = Replace Array Subset(array=w736, new element=w733, index (row)=8, index (col)=0) -> (w732:dbl[][])
      }
      event "2D Picture 82": Mouse Down {
        n377 = event-data() -> ("Button"=w744:u16)  [unwired: 1 in]
        n378 = To Unsigned Byte Integer(number=w744) -> (unsigned 8bit integer=w740:u8)
        n379 = call "Untitled 5 (SubVI).vi"("Button"=w744) -> ("new picture"=→"2D Picture 82":picture)  [unwired: 10 in]
        n380 = Replace Array Subset(array=w743, new element=w740, index (row)=8, index (col)=1) -> (w739:dbl[][])
      }
      event "2D Picture 83": Mouse Down {
        n381 = event-data() -> ("Button"=w751:u16)  [unwired: 1 in]
        n382 = To Unsigned Byte Integer(number=w751) -> (unsigned 8bit integer=w747:u8)
        n383 = call "Untitled 5 (SubVI).vi"("Button"=w751) -> ("new picture"=→"2D Picture 83":picture)  [unwired: 10 in]
        n384 = Replace Array Subset(array=w750, new element=w747, index (row)=8, index (col)=2) -> (w746:dbl[][])
      }
      event "2D Picture 84": Mouse Down {
        n385 = event-data() -> ("Button"=w758:u16)  [unwired: 1 in]
        n386 = To Unsigned Byte Integer(number=w758) -> (unsigned 8bit integer=w754:u8)
        n387 = call "Untitled 5 (SubVI).vi"("Button"=w758) -> ("new picture"=→"2D Picture 84":picture)  [unwired: 10 in]
        n388 = Replace Array Subset(array=w757, new element=w754, index (row)=8, index (col)=3) -> (w753:dbl[][])
      }
      event "2D Picture 85": Mouse Down {
        n389 = event-data() -> ("Button"=w765:u16)  [unwired: 1 in]
        n390 = To Unsigned Byte Integer(number=w765) -> (unsigned 8bit integer=w761:u8)
        n391 = call "Untitled 5 (SubVI).vi"("Button"=w765) -> ("new picture"=→"2D Picture 85":picture)  [unwired: 10 in]
        n392 = Replace Array Subset(array=w764, new element=w761, index (row)=8, index (col)=4) -> (w760:dbl[][])
      }
      event "2D Picture 86": Mouse Down {
        n393 = event-data() -> ("Button"=w772:u16)  [unwired: 1 in]
        n394 = To Unsigned Byte Integer(number=w772) -> (unsigned 8bit integer=w768:u8)
        n395 = call "Untitled 5 (SubVI).vi"("Button"=w772) -> ("new picture"=→"2D Picture 86":picture)  [unwired: 10 in]
        n396 = Replace Array Subset(array=w771, new element=w768, index (row)=8, index (col)=5) -> (w767:dbl[][])
      }
      event "2D Picture 87": Mouse Down {
        n397 = event-data() -> ("Button"=w779:u16)  [unwired: 1 in]
        n398 = To Unsigned Byte Integer(number=w779) -> (unsigned 8bit integer=w775:u8)
        n399 = call "Untitled 5 (SubVI).vi"("Button"=w779) -> ("new picture"=→"2D Picture 87":picture)  [unwired: 10 in]
        n400 = Replace Array Subset(array=w778, new element=w775, index (row)=8, index (col)=6) -> (w774:dbl[][])
      }
      event "2D Picture 88": Mouse Down {
        n401 = event-data() -> ("Button"=w786:u16)  [unwired: 1 in]
        n402 = To Unsigned Byte Integer(number=w786) -> (unsigned 8bit integer=w782:u8)
        n403 = call "Untitled 5 (SubVI).vi"("Button"=w786) -> ("new picture"=→"2D Picture 88":picture)  [unwired: 10 in]
        n404 = Replace Array Subset(array=w785, new element=w782, index (row)=8, index (col)=7) -> (w781:dbl[][])
      }
      event "2D Picture 89": Mouse Down {
        n405 = event-data() -> ("Button"=w793:u16)  [unwired: 1 in]
        n406 = To Unsigned Byte Integer(number=w793) -> (unsigned 8bit integer=w789:u8)
        n407 = call "Untitled 5 (SubVI).vi"("Button"=w793) -> ("new picture"=→"2D Picture 89":picture)  [unwired: 10 in]
        n408 = Replace Array Subset(array=w792, new element=w789, index (row)=8, index (col)=8) -> (w788:dbl[][])
      }
      event "2D Picture 90": Mouse Down {
        n409 = event-data() -> ("Button"=w800:u16)  [unwired: 1 in]
        n410 = To Unsigned Byte Integer(number=w800) -> (unsigned 8bit integer=w796:u8)
        n411 = call "Untitled 5 (SubVI).vi"("Button"=w800) -> ("new picture"=→"2D Picture 90":picture)  [unwired: 10 in]
        n412 = Replace Array Subset(array=w799, new element=w796, index (row)=8, index (col)=9) -> (w795:dbl[][])
      }
      event "2D Picture 91": Mouse Down {
        n413 = event-data() -> ("Button"=w807:u16)  [unwired: 1 in]
        n414 = To Unsigned Byte Integer(number=w807) -> (unsigned 8bit integer=w803:u8)
        n415 = call "Untitled 5 (SubVI).vi"("Button"=w807) -> ("new picture"=→"2D Picture 91":picture)  [unwired: 10 in]
        n416 = Replace Array Subset(array=w806, new element=w803, index (row)=9, index (col)=0) -> (w802:dbl[][])
      }
      event "2D Picture 92": Mouse Down {
        n417 = event-data() -> ("Button"=w814:u16)  [unwired: 1 in]
        n418 = To Unsigned Byte Integer(number=w814) -> (unsigned 8bit integer=w810:u8)
        n419 = call "Untitled 5 (SubVI).vi"("Button"=w814) -> ("new picture"=→"2D Picture 92":picture)  [unwired: 10 in]
        n420 = Replace Array Subset(array=w813, new element=w810, index (row)=9, index (col)=1) -> (w809:dbl[][])
      }
      event "2D Picture 93": Mouse Down {
        n421 = event-data() -> ("Button"=w821:u16)  [unwired: 1 in]
        n422 = To Unsigned Byte Integer(number=w821) -> (unsigned 8bit integer=w817:u8)
        n423 = call "Untitled 5 (SubVI).vi"("Button"=w821) -> ("new picture"=→"2D Picture 93":picture)  [unwired: 10 in]
        n424 = Replace Array Subset(array=w820, new element=w817, index (row)=9, index (col)=2) -> (w816:dbl[][])
      }
      event "2D Picture 94": Mouse Down {
        n425 = event-data() -> ("Button"=w828:u16)  [unwired: 1 in]
        n426 = To Unsigned Byte Integer(number=w828) -> (unsigned 8bit integer=w824:u8)
        n427 = call "Untitled 5 (SubVI).vi"("Button"=w828) -> ("new picture"=→"2D Picture 94":picture)  [unwired: 10 in]
        n428 = Replace Array Subset(array=w827, new element=w824, index (row)=9, index (col)=3) -> (w823:dbl[][])
      }
      event "2D Picture 95": Mouse Down {
        n429 = event-data() -> ("Button"=w835:u16)  [unwired: 1 in]
        n430 = To Unsigned Byte Integer(number=w835) -> (unsigned 8bit integer=w831:u8)
        n431 = call "Untitled 5 (SubVI).vi"("Button"=w835) -> ("new picture"=→"2D Picture 95":picture)  [unwired: 10 in]
        n432 = Replace Array Subset(array=w834, new element=w831, index (row)=9, index (col)=4) -> (w830:dbl[][])
      }
      event "2D Picture 96": Mouse Down {
        n433 = event-data() -> ("Button"=w842:u16)  [unwired: 1 in]
        n434 = To Unsigned Byte Integer(number=w842) -> (unsigned 8bit integer=w838:u8)
        n435 = call "Untitled 5 (SubVI).vi"("Button"=w842) -> ("new picture"=→"2D Picture 96":picture)  [unwired: 10 in]
        n436 = Replace Array Subset(array=w841, new element=w838, index (row)=9, index (col)=5) -> (w837:dbl[][])
      }
      event "2D Picture 97": Mouse Down {
        n437 = event-data() -> ("Button"=w849:u16)  [unwired: 1 in]
        n438 = To Unsigned Byte Integer(number=w849) -> (unsigned 8bit integer=w845:u8)
        n439 = call "Untitled 5 (SubVI).vi"("Button"=w849) -> ("new picture"=→"2D Picture 97":picture)  [unwired: 10 in]
        n440 = Replace Array Subset(array=w848, new element=w845, index (row)=9, index (col)=6) -> (w844:dbl[][])
      }
      event "2D Picture 98": Mouse Down {
        n441 = event-data() -> ("Button"=w856:u16)  [unwired: 1 in]
        n442 = To Unsigned Byte Integer(number=w856) -> (unsigned 8bit integer=w852:u8)
        n443 = call "Untitled 5 (SubVI).vi"("Button"=w856) -> ("new picture"=→"2D Picture 98":picture)  [unwired: 10 in]
        n444 = Replace Array Subset(array=w855, new element=w852, index (row)=9, index (col)=7) -> (w851:dbl[][])
      }
      event "2D Picture 99": Mouse Down {
        n445 = event-data() -> ("Button"=w863:u16)  [unwired: 1 in]
        n446 = To Unsigned Byte Integer(number=w863) -> (unsigned 8bit integer=w859:u8)
        n447 = call "Untitled 5 (SubVI).vi"("Button"=w863) -> ("new picture"=→"2D Picture 99":picture)  [unwired: 10 in]
        n448 = Replace Array Subset(array=w862, new element=w859, index (row)=9, index (col)=8) -> (w858:dbl[][])
      }
      event "2D Picture 100": Mouse Down {
        n449 = event-data() -> ("Button"=w870:u16)  [unwired: 1 in]
        n450 = To Unsigned Byte Integer(number=w870) -> (unsigned 8bit integer=w866:u8)
        n451 = call "Untitled 5 (SubVI).vi"("Button"=w870) -> ("new picture"=→"2D Picture 100":picture)  [unwired: 10 in]
        n452 = Replace Array Subset(array=w869, new element=w866, index (row)=9, index (col)=9) -> (w865:dbl[][])
      }
    }
    n453 = Index Array(array=w141, index=0) -> (element=w132:i32)
    n454 = Index Array(array=w141, index=1) -> (element=w131:i32)
    n455 = Multiply(x=w132, y=w131) -> (x*y=w135:i32)
    n456 = for {
      N: w132 -> [_]
      tunnel: w131 -> [w151]
      tunnel: w130 -> [w150] mode=indexing
      tunnel: w138 -> [w149] mode=indexing
      shift-right: [w148] -> w136
      shift-left: 0 -> [w147]
      n457 = for {
        N: w151 -> [_]
        tunnel: w150 -> [w155] mode=indexing
        tunnel: w149 -> [w154] mode=indexing
        shift-right: [w152] -> w148
        shift-left: w147 -> [w153]
        n458 = case shown="False" w155 {
          tunnel: w154 -> [w158 w167]
          tunnel: w153 -> [w157 w165]
          tunnel: [w156 w164] -> w152
          frame False {
            n459 = Not Equal?(x=w158, y=1.0) -> (x != y?=w162:bool)
            n460 = Select(t=1.0, s=w162, f=0.0) -> (s? t:f=w163:dbl)
            n461 = Add(x=w157, y=w163) -> (x+y=w156:dbl)
          }
          frame True {
            n462 = Equal?(x=w167, y=1.0) -> (x = y?=w171:bool)
            n463 = Select(t=1.0, s=w171, f=0.0) -> (s? t:f=w166:dbl)
            n464 = Add(x=w165, y=w166) -> (x+y=w164:dbl)
          }
        }
      }
    }
    n465 = Equal?(x=w136, y=w135) -> (x = y?=w134:bool)
    n466 = case shown="True" w134 {
      tunnel: [FALSE ("true") w144] -> w133
      frame False {
      }
      frame True {
        n467 = One Button Dialog(message="Congrats! You have finished fishrcross!", button name ("OK")="Cool!") -> (true=w144:bool)
      }
    }
  }
